vi "Stepper Driver.vi"(10 "Stepper Tick":T1, 11 "Stepper Action":T2) -> ()   [LabVIEW 2018]
uses:
  AFM Controls/FPGA/Stepper_Commands.ctl
  AFM Controls/FPGA/Stepper_Parameters.ctl
  <vilib>/rvi/eio/common/nirviEmuTemplateMethod_errors.vi
  <vilib>/eio/EIONode/EIONode.xnode
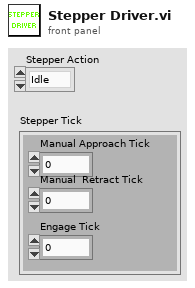
[diagram p1: front panel]
types:
  T1 = typedef "Stepper_Parameters.ctl" = cluster{"Engage Tick":i32, "Manual Approach Tick":i32, "Manual  Retract Tick":i32}
  T2 = typedef "Stepper_Commands.ctl" = enum16{"Idle", "Hold", "Manual Approach", "Manual Retract", "Engage", "Release"}
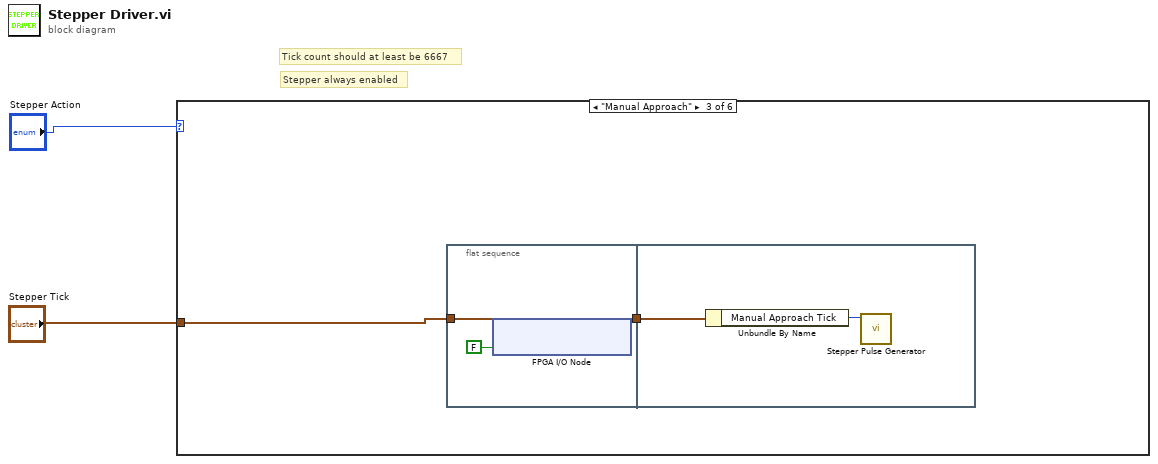
[diagram p0: block diagram]
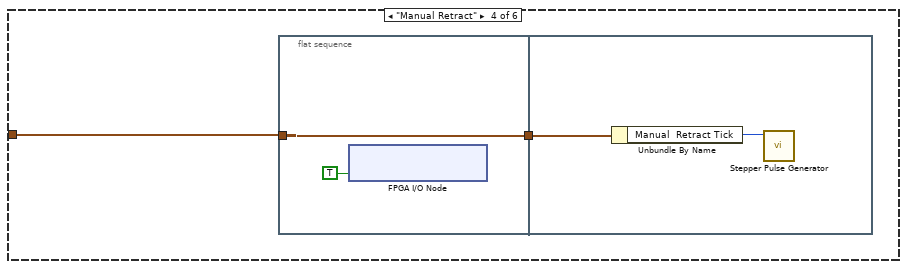
[diagram p4: hidden frame]
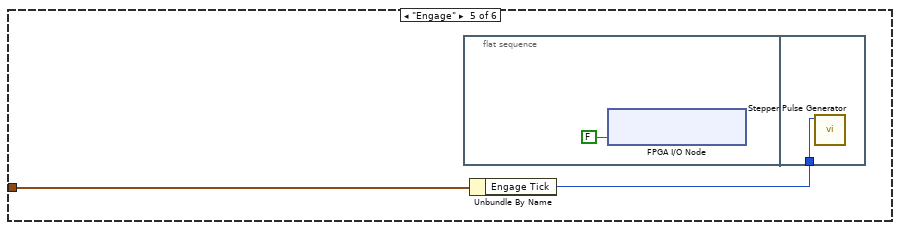
[diagram p5: hidden frame]
diagram:
  # "Stepper always enabled"
  # "Tick count should at least be 6667"
  n1 = case shown="\"Manual Approach\"" "Stepper Action" {
    tunnel: "Stepper Tick" -> [_ _ w4 w10 w16 _]
    frame "Idle" {
    }
    frame "Hold", Default {
    }
    frame "Manual Approach" {
      n2 = flat-sequence {
        tunnel: w4 -> [w6]
        tunnel: [w6] -> w3
        tunnel: w3 -> [w8]
        frame #0 {
          n3 = xnode "FPGA I/O Node"("ConnectorA/DIO1"=FALSE ("Connector0/DIO2")) -> ()  [unwired: 1 in, 1 out]
        }
        frame #1 {
          n4 = Unbundle By Name(w8) -> ("Manual Approach Tick"=w7:i32)
          n5 = call "Stepper Pulse Generator.vi"("Tick Count"=w7) -> ()  [unwired: 11 in]
        }
      }
    }
    frame "Manual Retract" {
      n6 = flat-sequence {
        tunnel: w10 -> [w12]
        tunnel: [w12] -> w9
        tunnel: w9 -> [w13]
        frame #0 {
          n7 = xnode "FPGA I/O Node"("ConnectorA/DIO1"=TRUE ("Connector0/DIO2")) -> ()  [unwired: 1 in, 1 out]
        }
        frame #1 {
          n8 = Unbundle By Name(w13) -> ("Manual  Retract Tick"=w14:i32)
          n9 = call "Stepper Pulse Generator.vi"("Tick Count"=w14) -> ()  [unwired: 11 in]
        }
      }
    }
    frame "Engage" {
      n10 = flat-sequence {
        tunnel: w15 -> [w18]
        frame #0 {
          n11 = xnode "FPGA I/O Node"("ConnectorA/DIO1"=FALSE ("Connector0/DIO2")) -> ()  [unwired: 1 in, 1 out]
        }
        frame #1 {
          n12 = call "Stepper Pulse Generator.vi"("Tick Count"=w18) -> ()  [unwired: 11 in]
        }
      }
      n13 = Unbundle By Name(w16) -> ("Engage Tick"=w15:i32)
    }
    frame "Release" {
    }
  }
